vi "Network Stream Module.vi"(8 "error in (no error)":errorcluster, 10 "Image In":T2, 11 "Operation":T1) -> (0 "error out":errorcluster)   [LabVIEW 2013]
uses:
  <vilib>/vision/Image Controls.llb/IMAQ Image.ctl
  Network Stream Module Enum.ctl
  <vilib>/dex/Stream Element Allocation Mode.ctl
  <vilib>/ErrorRing/Error Ring.xnode
panel:
  in  "Target IP Address":string="localhost"
  out "reader url":string
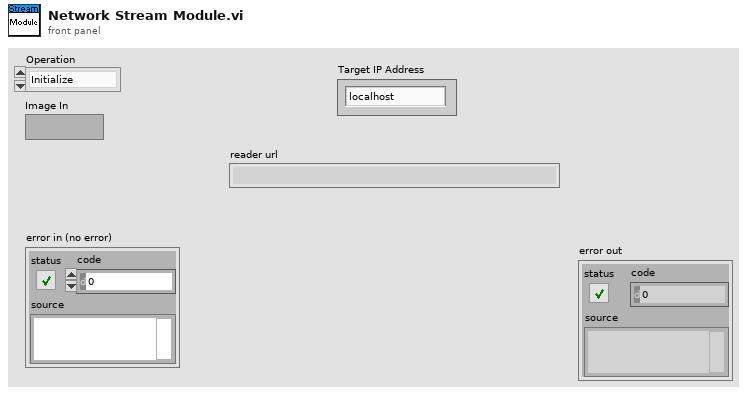
[diagram p1: front panel]
types:
  T1 = typedef "Network Stream Module Enum.ctl" = enum16{"Initialize", "Write", "Close"}
  T2 = typedef "IMAQ Image.ctl" = refnum<image>
  T3 = typedef "Stream Element Allocation Mode.ctl" = u32
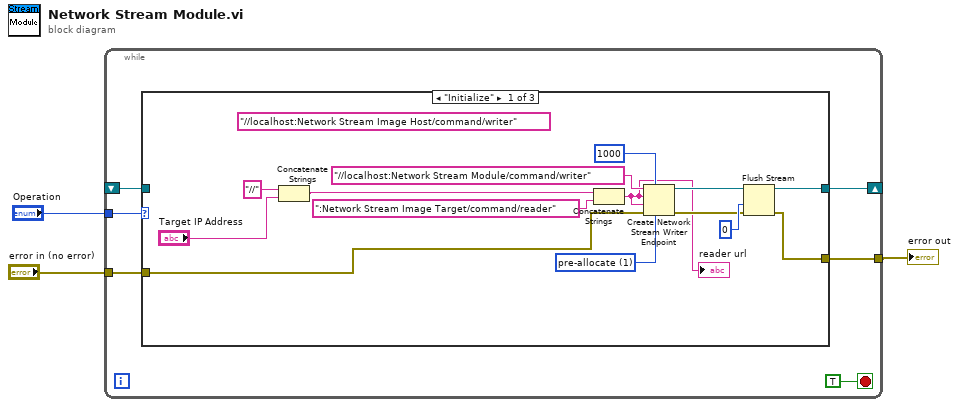
[diagram p0: block diagram]
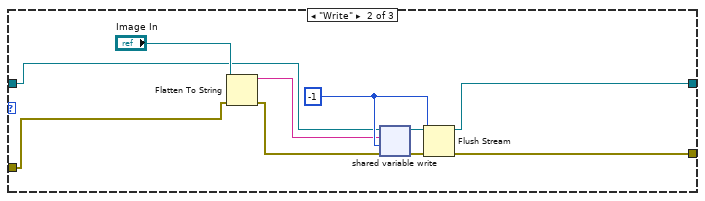
[diagram p2: hidden frame]
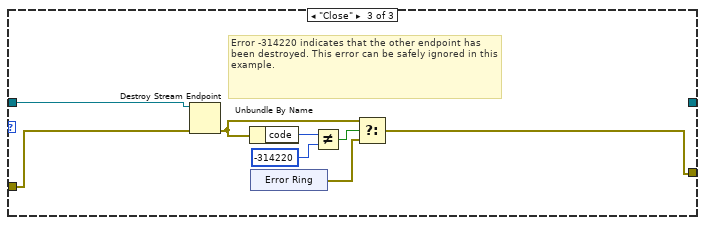
[diagram p3: hidden frame]
diagram:
  n1 = while {
    shift-right: [w8] -> _
    shift-left: _ -> [w6]
    tunnel: "error in (no error)" -> [w7]
    tunnel: [w5] -> w2
    tunnel: "Operation" -> [w4]
    stop <- TRUE stop-if-true
    n2 = case shown="\"Initialize\"" w4 {
      tunnel: [w12 w24 _] -> w8
      tunnel: w7 -> [w10 w28 w35]
      tunnel: w6 -> [_ w26 w41]
      tunnel: [w11 w25 w34] -> w5
      frame "Initialize" {
        (unwired) "//localhost:Network Stream Image Host/command/writer" ("writer name")
        w17 = T3 1 items=["allocate as needed", "pre-allocate"] ("element allocation mode")
        n3 = Concatenate Strings("//" ("reader url"), "Target IP Address") -> (w14:string)
        n4 = Concatenate Strings(w14, ":Network Stream Image Target/command/reader" ("reader url")) -> (w13:string)
        "reader url" <- w13
        n5 = Create Network Stream Writer Endpoint(6:w17, 7:1000 ("writer buffer size"), 8:w10, 9:w13, 10:w13, 11:"//localhost:Network Stream Module/command/writer" ("writer name")) -> (0:w18:errorcluster, 3:w19:refnum<k21>)  [unwired: 1 in]
        n6 = Flush Stream(8:w18, 9:0 ("timeout in ms (-1)"), 11:w19) -> (0:w11:errorcluster, 3:w12:refnum<k21>)  [unwired: 1 in, 1 out]
      }
      frame "Write" {
        w31 = -1 ("timeout in ms (-1)")
        n7 = Flatten To String(anything="Image In", error in (no error)=w28) -> (data string=w30:string, error out=w27:errorcluster)  [unwired: 2 in, 1 out]
        n8 = shared-variable-write(w26, w27, w30, w31) -> (w33:refnum<k21>, w32:errorcluster)  [unwired: 1 out]
        n9 = Flush Stream(8:w32, 9:w31, 11:w33) -> (0:w25:errorcluster, 3:w24:refnum<k21>)  [unwired: 1 in, 1 out]
      }
      frame "Close" {
        # "Error -314220 indicates that the other endpoint has been destroyed. This error can be safely ignored in this example."
        n10 = Destroy Stream Endpoint(8:w35, 11:w41) -> (0:w36:errorcluster)
        n11 = Unbundle By Name(w36) -> ("code"=w40:i32)
        n12 = xnode "Error Ring"() -> ("error out"=w37:errorcluster)
        n13 = Not Equal?(x=w40, y=-314220) -> (x != y?=w38:bool)
        n14 = Select(t=w36, s=w38, f=w37) -> (s? t:f=w34:errorcluster)
      }
    }
  }
  "error out" <- w2
